vi "PhysMon-Init Data File.vi"(0 "Path":path, 11 "error in (no error)":errorcluster) -> (12 "Notes":string[][](array[string]), 13 "Temp Data":cluster{timestamp, dbl}[](array[cluster]), 14 "HR Data":cluster{timestamp, dbl}[](array[cluster]), 15 "error out":errorcluster)   [LabVIEW 2020]
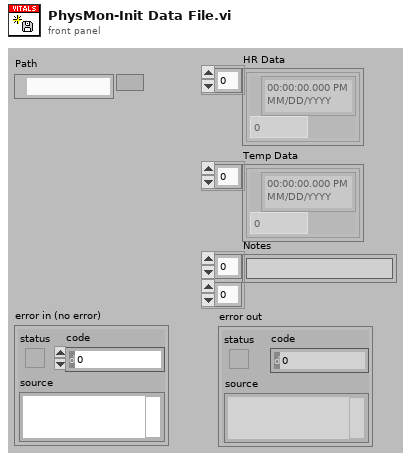
[diagram p1: front panel]
types:
  T1 = cluster{"seconds since 1Jan1904":timestamp, dbl}[]
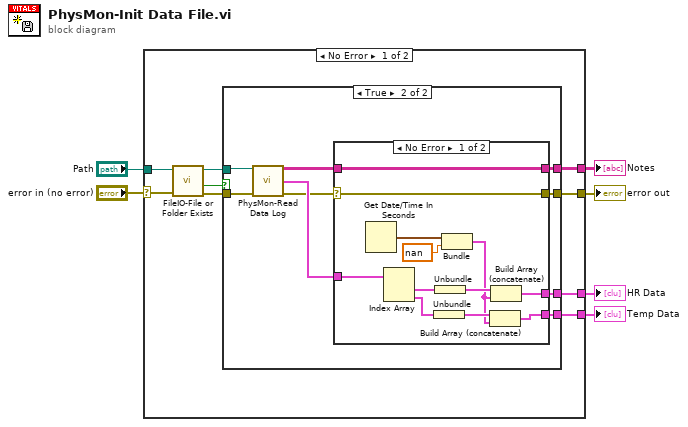
[diagram p0: block diagram]
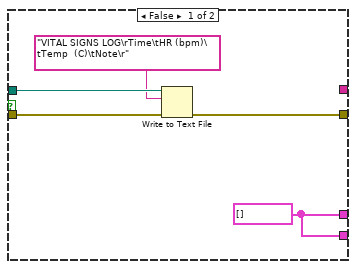
[diagram p2: hidden frame]
diagram:
  n1 = case shown="No Error" "error in (no error)" {
    selector: "error in (no error)" -> [w14 w43]
    tunnel: [w8 w43] -> w5
    tunnel: "Path" -> [w15 _]
    tunnel: [w10 _] -> w3
    tunnel: [w9 _] -> w2
    tunnel: [w7 _] -> w1
    frame No Error {
      n2 = call "FileIO-File or Folder Exists.vi"("error in (no error)"=w14, "path"=w15) -> ("error out"=w11:errorcluster, "Exists?"=w13:bool, "dup path"=w12:path)  [unwired: 6 in, 1 out]
      n3 = case shown="True" w13 {
        tunnel: w12 -> [w20 w28]
        tunnel: w11 -> [w19 w29]
        tunnel: [w18 w26] -> w10
        tunnel: [w18 w25] -> w9
        tunnel: [w17 w23] -> w8
        tunnel: [_ w21] -> w7
        frame False {
          w18 = cluster{timestamp, dbl}[] [] ("HR Data")
          n4 = Write to Text File(file (use dialog)=w20, text="VITAL SIGNS LOG\rTime\tHR (bpm)\tTemp  (C)\tNote\r", error in=w19) -> (error out=w17:errorcluster)  [unwired: 1 in, 2 out]
        }
        frame True {
          n5 = call "PhysMon-Read Data Log.vi"("Path"=w28, "error in (no error)"=w29) -> ("Notes"=w22:string[][], "Vital Signs Graph"=w27:cluster{"HR Data":cluster{timestamp, dbl}[]}[], "error out"=w24:errorcluster)  [unwired: 11 in]
          n6 = case shown="No Error" w24 {
            selector: w24 -> [w36 w42]
            tunnel: w27 -> [w41 _]
            tunnel: [w34 _] -> w26
            tunnel: [w33 _] -> w25
            tunnel: [w36 w42] -> w23
            tunnel: w22 -> [w30 _]
            tunnel: [w30 _] -> w21
            frame No Error {
              n7 = Get Date/Time In Seconds() -> (seconds since 1Jan1904=w32:timestamp)
              n8 = Index Array(array=w41) -> (element #1=w40:cluster{"HR Data":cluster{timestamp, dbl}[]}, element #2=w39:cluster{"HR Data":cluster{timestamp, dbl}[]})  [unwired: 2 in]
              n9 = Unbundle(w39) -> ("HR Data"=w37:cluster{timestamp, dbl}[])
              n10 = Unbundle(w40) -> ("HR Data"=w38:cluster{timestamp, dbl}[])
              n11 = Bundle("seconds since 1Jan1904"=w32, nan) -> (w31:cluster{"seconds since 1Jan1904":timestamp, dbl})  [unwired: 1 in]
              n12 = Build Array (concatenate)(w37, w31) -> (w33:T1)
              n13 = Build Array (concatenate)(w38, w31) -> (w34:T1)
            }
            frame Error {
            }
          }
        }
      }
    }
    frame Error {
    }
  }
  "error out" <- w5
  "HR Data" <- w3
  "Temp Data" <- w2
  "Notes" <- w1
